vi "Close File.vi"(8 "error in":errorcluster, 10 "File Refnum":variant, 11 "CSV File in":refnum<class "CSV File.lvclass">) -> (0 "error out":errorcluster, 3 "CSV File out":refnum<class "CSV File.lvclass">)   [LabVIEW 2021, in "CSV File.lvclass"]
doc: "This vi helps to close CSV file."
uses:
  CSV File.lvclass
  File Abstract Class/File Abstract.lvclass
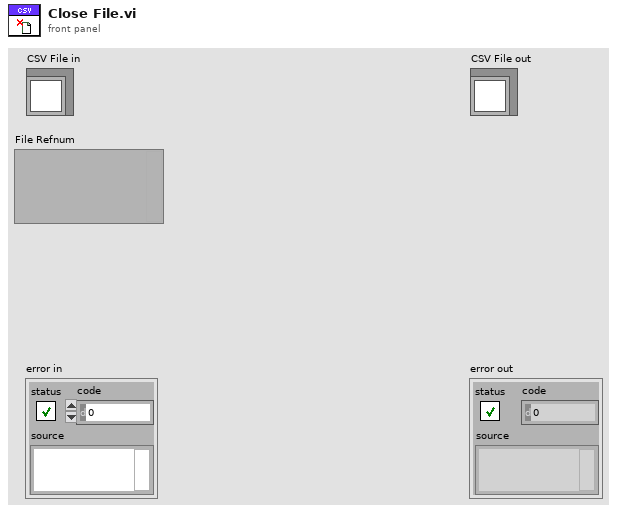
[diagram p1: front panel]
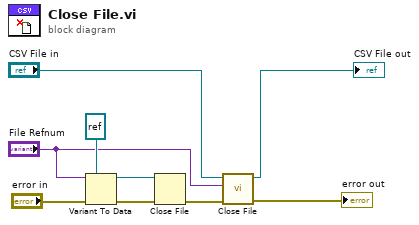
[diagram p0: block diagram]
diagram:
  n1 = Variant To Data(error in="error in", type=refnum<file> refnum ("CSV Refnum"), Variant="File Refnum") -> (data=w5:refnum<file>, error out=w4:errorcluster)
  n2 = Close File(refnum=w5, error in=w4) -> (error out=w7:errorcluster)  [unwired: 1 out]
  n3 = call-parent "Close File.vi"("error in (no error)"=w7, "File Refnum"="File Refnum", "File Manager in"="CSV File in") -> ("error out"=→"error out":errorcluster, "File Manager out"=→"CSV File out":refnum<class "CSV File.lvclass">)  [unwired: 7 in]
